vi "公式节点.vi"() -> ()   [LabVIEW 2015]
panel:
  out "Waveform Graph 4":dbl[](graph)
  out "Waveform Graph 3":dbl[](graph)
  out "Waveform Graph 2":dbl[](graph)
  out "Waveform Graph 1":dbl[](graph)
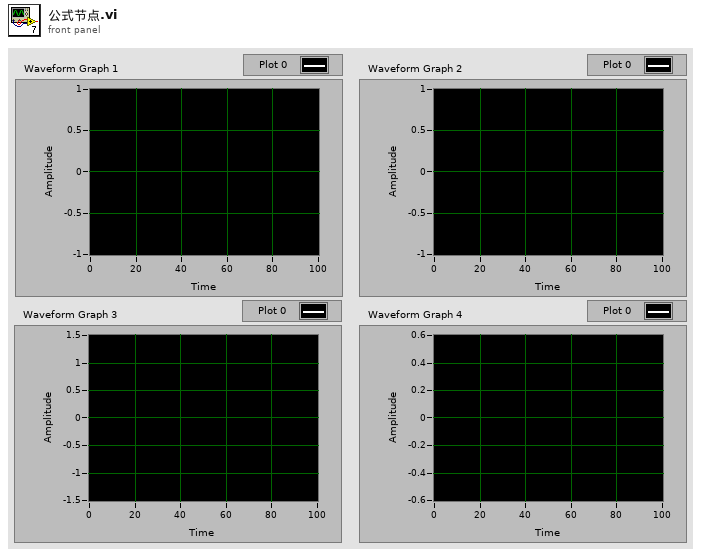
[diagram p1: front panel]
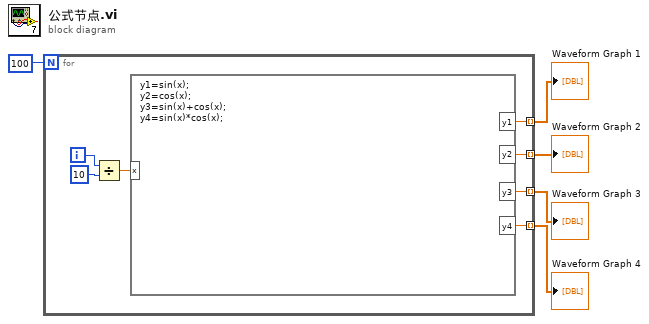
[diagram p0: block diagram]
diagram:
  n1 = for {
    N: 100 -> [_]
    tunnel: [w9] -> w4 mode=indexing
    tunnel: [w8] -> w3 mode=indexing
    tunnel: [w7] -> w2 mode=indexing
    tunnel: [w6] -> w1 mode=indexing
    i -> [w12]
    n2 = Divide(x=w12, y=10) -> (x/y=w10:dbl)
    n3 = formula code="y1=sin(x);\ny2=cos(x);\ny3=sin(x)+cos(x);\ny4=sin(x)*cos(x);"("x"=w10) -> ("y1"=w9:dbl, "y2"=w8:dbl, "y3"=w7:dbl, "y4"=w6:dbl)
  }
  "Waveform Graph 3" <- w2
  "Waveform Graph 4" <- w1
  "Waveform Graph 2" <- w3
  "Waveform Graph 1" <- w4
